vi "GW_Display_data.vi"(8 "error in (no error)":errorcluster, 11 "DBlink":string="Driver={ODBC Driver 17 for SQL Server};Server=localhost\\SQLEXPRESS;Database=ZDX201;UID=labview;PWD=Dsa@54137926") -> (0 "error out":errorcluster, 3 "Workplace":T1(array[cluster])=[{"id"=1, "站點位置"="上料", "glue_data_id"="{C553317C-B37B-43B8-A6AD-52622C31A48F}", "更新時間"="2022/7/5 下午 02:13:38"}, {"id"=2, "站點位置"="移動中_離開上料", "glue_data_id"="", "更新時間"="2022/7/5 下午 01:16:28"}, {"id"=3, "站點位置"="散熱膏", "glue_data_id"="", "更新時間"="2022/7/5 下午 01:16:28"}, {"id"=4, "站點位置"="移動中_離開散熱膏", "glue_data_id"="", "更新時間"="2022/7/5 下午 01:16:28"}, {"id"=5, "站點位置"="檢測一", "glue_data_id"="", "更新時間"="2022/7/5 下午 01:16:28"}, {"id"=6, "站點位置"="移動中_離開檢測一", "glue_data_id"="", "更新時間"="2022/7/5 下午 01:16:28"}, {"id"=7, "站點位置"="密封一", "glue_data_id"="", "更新時間"="2022/7/5 下午 01:16:28"}, {"id"=8, "站點位置"="移動中_離開密封一", "glue_data_id"="", "更新時間"="2022/7/5 下午 01:16:28"}, {"id"=9, "站點位置"="密封二", "glue_data_id"="", "更新時間"="2022/7/5 下午 01:16:28"}, {"id"=10, "站點位置"="移動中_離開密封二", "glue_data_id"="", "更新時間"="2022/7/5 下午 01:16:28"}, {"id"=11, "站點位置"="檢測二", "glue_data_id"="", "更新時間"="2022/7/5 下午 01:16:28"}, {"id"=12, "站點位置"="移動中_離開檢測二", "glue_data_id"="", "更新時間"="2022/7/5 下午 01:16:28"}, {"id"=13, "站點位置"="待料站", "glue_data_id"="", "更新時間"="2022/7/5 下午 01:16:28"}, {"id"=14, "站點位置"="手臂上", "glue_data_id"="", "更新時間"="2022/7/5 下午 01:16:28"}, {"id"=15, "站點位置"="組合R", "glue_data_id"="", "更新時間"="2022/7/5 下午 01:16:28"}, {"id"=16, "站點位置"="組合L", "glue_data_id"="", "更新時間"="2022/7/5 下午 01:16:28"}, {"id"=17, "站點位置"="NG下料", "glue_data_id"="", "更新時間"="2022/7/5 下午 01:16:28"}])   [LabVIEW 2019]
uses:
  <vilib>/addons/database/Connection.llb/DB Tools Open Connec (String).vi
  <vilib>/addons/database/Connection.llb/Conn Execute.vi
  <vilib>/addons/database/Recordset.llb/Rec Fetch Recordset Data (R).vi
  <vilib>/addons/database/Recordset.llb/Rec Destroy - Connection.vi
  <vilib>/addons/database/_DB Variant To Data/Database Variant To Data.xnode
  <vilib>/addons/database/NI_Database_API.lvlib
panel:
  out "查詢結果":string="/****** SSMS 中 SelectTopNRows 命令的指令碼  ******/\nSELECT TOP (1000) [id]\n      ,[name]\n      ,[glue_data_id]\n      ,[update_time]\n  FROM [ZDX201].[dbo].[glue_workspace]"
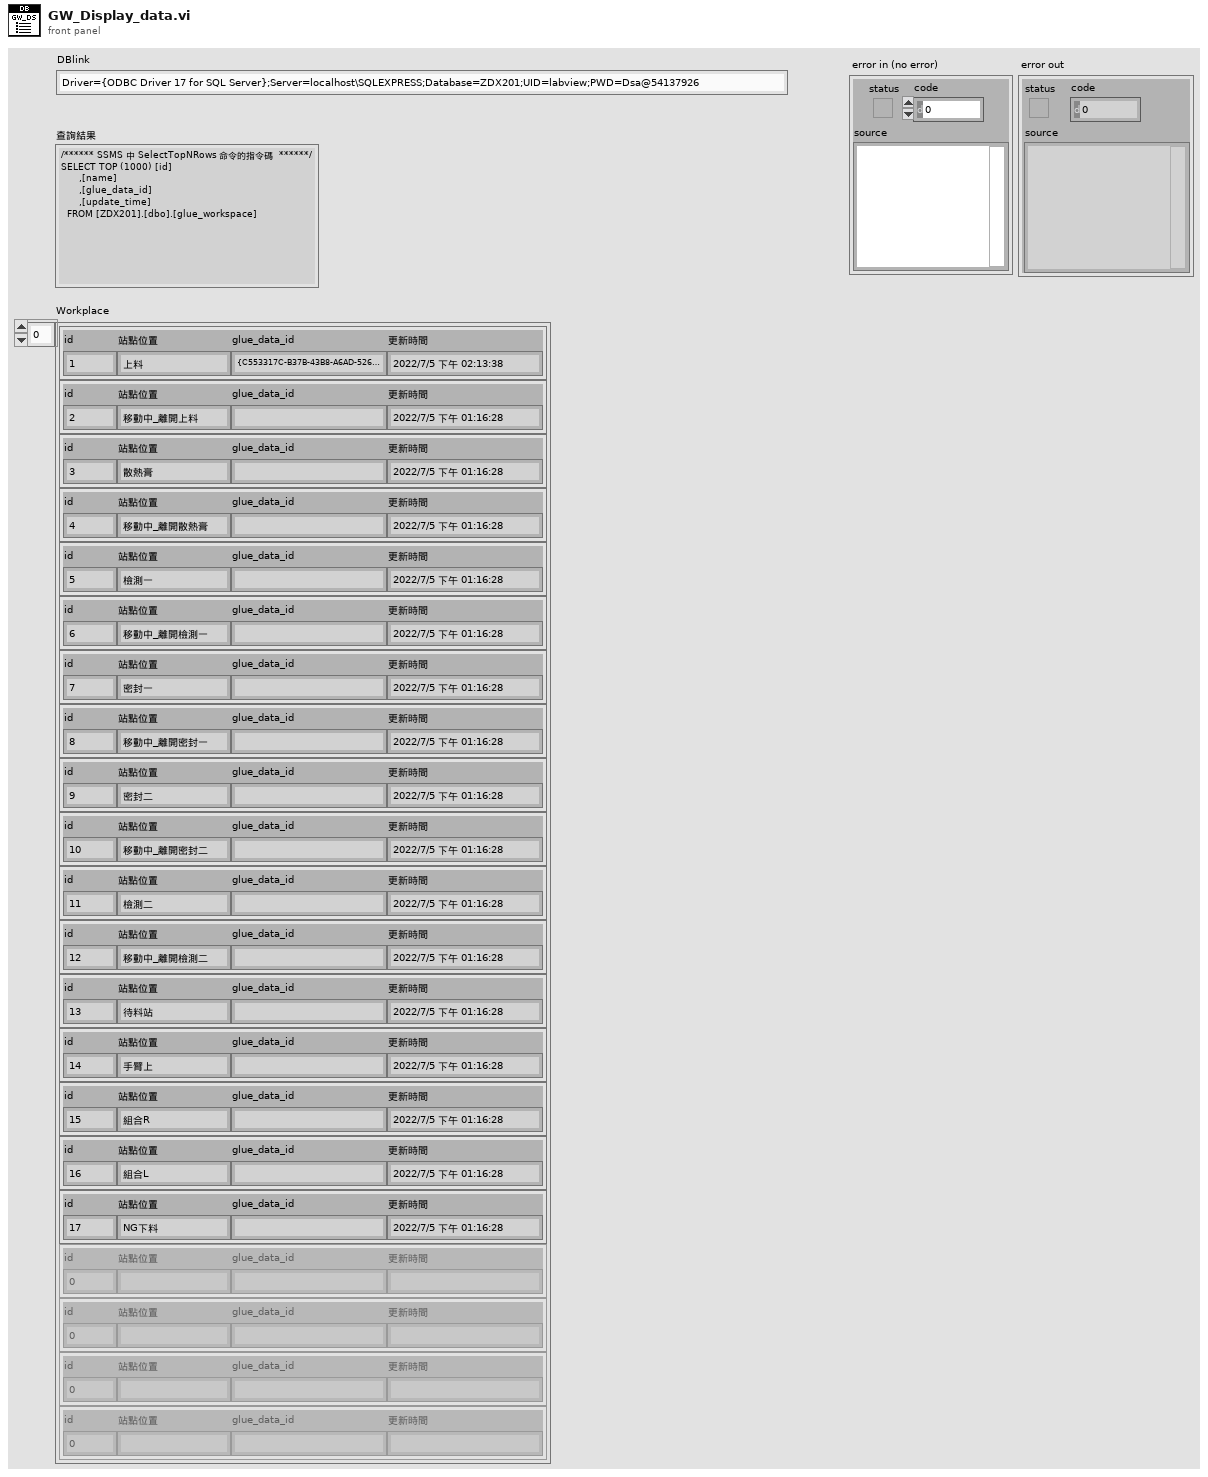
[diagram p1: front panel]
types:
  T1 = cluster{"id":i32, "站點位置":string, "glue_data_id":string, "更新時間":string}[]
  T2 = typedef "NI_Database_API.lvlib/Conn ObjectReference.ctl" = refnum<k1>
  T3 = typedef "NI_Database_API.lvlib/Rec ObjectReference.ctl" = refnum<k1>
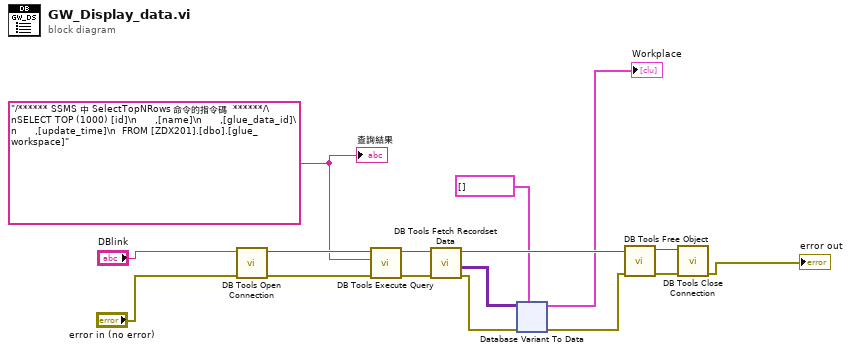
[diagram p0: block diagram]
diagram:
  w6 = "/****** SSMS 中 SelectTopNRows 命令的指令碼  ******/\nSELECT TOP (1000) [id]\n      ,[name]\n      ,[glue_data_id]\n      ,[update_time]\n  FROM [ZDX201].[dbo].[glue_workspace]"
  n1 = call-poly <vilib>:"DB Tools Open Connection.vi"("error in (no error)"="error in (no error)", "connection information"="DBlink") -> ("error out"=w16:errorcluster, "connection reference"=w15:T2)  [unwired: 6 in]
  n2 = call-poly <vilib>:"DB Tools Execute Query.vi"("error in (no error)"=w16, "SQL query"=w6, "connection reference"=w15) -> ("error out"=w13:errorcluster, "recordset reference"=w14:T3)  [unwired: 5 in]
  n3 = call-poly <vilib>:"DB Tools Fetch Recordset Data.vi"("error in (no error)"=w13, "recordset reference"=w14) -> ("error out"=w8:errorcluster, "recordset data"=w7:variant[][], "recordset reference out"=w9:T3)  [unwired: 3 in]
  n4 = xnode "Database Variant To Data"("database variant"=w7, "error in (no error)"=w8, "type"=T1 [] ("Workplace")) -> ("data"=→"Workplace":T1, "error out"=w10:errorcluster)
  n5 = call-poly <vilib>:"DB Tools Free Object.vi"("error in (no error)"=w10, "recordset reference"=w9) -> ("error out"=w11:errorcluster, "connection reference"=w12:T2)  [unwired: 8 in]
  n6 = call <vilib>:"DB Tools Close Connection.vi"("error in (no error)"=w11, "connection reference"=w12) -> ("error out"=→"error out":errorcluster)  [unwired: 5 in]
  "查詢結果" <- w6
